vi "pan2txt.vi"(5 "seconds since 1Jan1904":timestamp, 6 "started":timestamp, 7 "stop button":refnum<vi>) -> ()   [LabVIEW 2010]
uses:
  Global 2.vi
panel:
  out "last mod":timestamp
  out "volume path":path
  out "Array":string[](array[string])
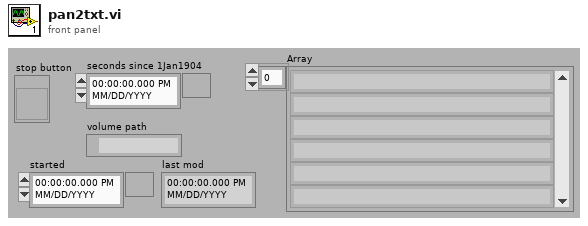
[diagram p1: front panel]
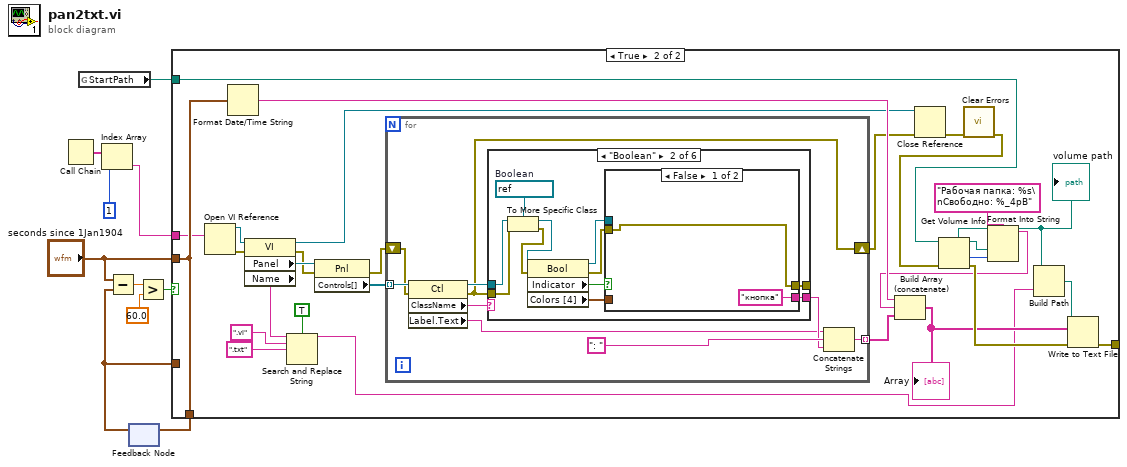
[diagram p0: block diagram]
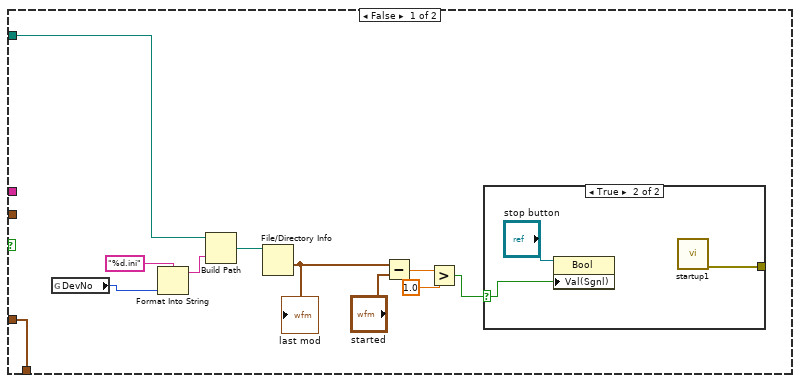
[diagram p2: hidden frame]
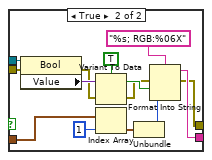
[diagram p5: hidden frame]
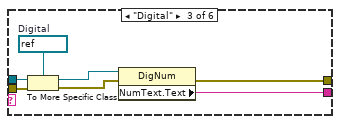
[diagram p6: hidden frame]
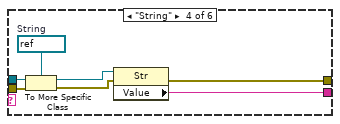
[diagram p7: hidden frame]
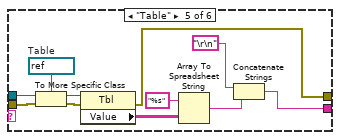
[diagram p8: hidden frame]
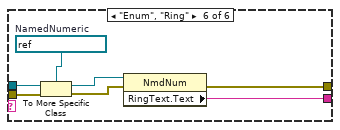
[diagram p9: hidden frame]
diagram:
  n1 = Call Chain() -> (call chain=w3:string[])
  n2 = global read "Global 2.vi" "StartPath"() -> (w1:path)
  n3 = Index Array(array=w3, index=1) -> (element=w2:string)
  n4 = feedback #1() -> (w5:timestamp)  [unwired: 1 in]
  n5 = Subtract(x="seconds since 1Jan1904", y=w5) -> (x-y=w10:dbl)
  n6 = Greater?(x=w10, y=60.0) -> (0:w8:bool)
  n7 = case shown="True" w8 {
    tunnel: "seconds since 1Jan1904" -> [_ w43]
    tunnel: [w21 w43] -> w6
    tunnel: w5 -> [w21 _]
    tunnel: [_ w41] -> _
    tunnel: w2 -> [_ w27]
    tunnel: w1 -> [w11 w25]
    frame False {
      n8 = global read "Global 2.vi" "DevNo"() -> (w20:i32)
      n9 = Format Into String(format string="%d.ini", w20) -> (resulting string=w18:string)  [unwired: 2 in, 1 out]
      n10 = Build Path(base path=w11, name or relative path=w18) -> (appended path=w17:path)
      n11 = File/Directory Info(path=w17) -> (last mod=w16:timestamp)  [unwired: 1 in, 6 out]
      "last mod" <- w16
      n12 = Subtract(x=w16, y="started") -> (x-y=w14:dbl)
      n13 = Greater?(x=w14, y=1.0) -> (0:w12:bool)
      n14 = case shown="True" w12 {
        selector: w12 -> [_ w23]
        tunnel: [_ w22] -> _
        frame False {
        }
        frame True {
          n15 = property class="Bool"(reference="stop button", "Val(Sgnl)"=w23) -> ()  [unwired: 1 in, 2 out]
          n16 = call "startup1.vi"() -> ("error out"=w22:errorcluster)  [unwired: 7 in]
        }
      }
    }
    frame True {
      n17 = Open VI Reference(vi path=w27) -> (vi reference=w50:refnum<vi>, error out=w53:errorcluster)  [unwired: 5 in]
      n18 = Format Date/Time String(seconds (now)=w43) -> (date/time string=w38:string)  [unwired: 2 in]
      n19 = property class="VI"(reference=w50, error in=w53) -> (reference out=w35:refnum<vi>, error out=w49:errorcluster, "Panel"=w52:refnum<vi>, "Name"=w32:string)
      n20 = Search and Replace String(case sensitive?=TRUE ("ignore case? (F)"), input string=w32, search string=".vi", replace string=".txt" ("replace string (\"\")")) -> (result string=w28:string)  [unwired: 4 in, 3 out]
      n21 = property class="Pnl"(reference=w52, error in=w49) -> (error out=w48:errorcluster, "Controls[]"=w51:refnum<vi>[])  [unwired: 1 out]
      n22 = for {
        tunnel: w51 -> [w62] mode=indexing
        tunnel: [w61] -> w44 mode=indexing
        shift-right: [w54] -> w36
        shift-left: w48 -> [w60]
        n23 = property class="Ctl"(reference=w62, error in=w60) -> (reference out=w57:refnum<vi>, error out=w54:errorcluster, "ClassName"=w58:string, "Label.Text"=w55:string)
        n24 = case shown="\"Boolean\"" w58 {
          selector: w58 -> [w64 _ _ _ _ _]
          tunnel: w57 -> [_ w75 w97 w104 w115 w122]
          tunnel: [w64 w73 w95 w102 w107 w120] -> w56
          tunnel: w54 -> [w63 w72 w94 w101 w111 w119]
          tunnel: [w63 w65 w92 w99 w106 w117] -> _
          frame "Any", Default {
          }
          frame "Boolean" {
            w74 = refnum<vi> refnum  # Boolean
            n25 = To More Specific Class(target class=w74, reference=w75, error in=w72) -> (specific class reference=w71:refnum<vi>, error out=w69:errorcluster)
            n26 = property class="Bool"(reference=w71, error in=w69) -> (reference out=w68:refnum<vi>, error out=w67:errorcluster, "Indicator"=w70:bool, "Colors [4]"=w66:cluster{u32, u32}[])
            n27 = case shown="False" w70 {
              tunnel: w68 -> [_ w91]
              tunnel: ["кнопка" w84] -> w73
              tunnel: w67 -> [w77 w82]
              tunnel: w66 -> [_ w81]
              tunnel: [w77 w80] -> w65
              frame False {
              }
              frame True {
                n28 = property class="Bool"(reference=w91, error in=w82) -> (error out=w79:errorcluster, "Value"=w88:variant)  [unwired: 1 out]
                n29 = Variant To Data(error in=w79, Variant=w88, type=TRUE) -> (error out=w78:errorcluster, data=w86:bool)
                n30 = Index Array(array=w81, index=1) -> (element=w90:cluster{u32, u32})
                n31 = Unbundle(w90) -> (w85:u32)  [unwired: 1 out]
                n32 = Format Into String(format string="%s; RGB:%06X", error in=w78, w86, w85) -> (resulting string=w84:string, error out=w80:errorcluster)  [unwired: 1 in]
              }
            }
          }
          frame "Digital" {
            w98 = refnum<vi> refnum  # Digital
            n33 = To More Specific Class(target class=w98, reference=w97, error in=w94) -> (specific class reference=w96:refnum<vi>, error out=w93:errorcluster)
            n34 = property class="DigNum"(reference=w96, error in=w93) -> (error out=w92:errorcluster, "NumText.Text"=w95:string)  [unwired: 1 out]
          }
          frame "String" {
            w105 = refnum<vi> refnum  # String
            n35 = To More Specific Class(target class=w105, reference=w104, error in=w101) -> (specific class reference=w103:refnum<vi>, error out=w100:errorcluster)
            n36 = property class="Str"(reference=w103, error in=w100) -> (error out=w99:errorcluster, "Value"=w102:string)  [unwired: 1 out]
          }
          frame "Table" {
            w116 = refnum<vi> refnum  # Table
            n37 = To More Specific Class(target class=w116, reference=w115, error in=w111) -> (specific class reference=w114:refnum<vi>, error out=w110:errorcluster)
            n38 = property class="Tbl"(reference=w114, error in=w110) -> (error out=w106:errorcluster, "Value"=w113:string[][])  [unwired: 1 out]
            n39 = Array To Spreadsheet String(array=w113, 3:"%s" ("format string")) -> (spreadsheet string=w109:string)  [unwired: 1 in]
            n40 = Concatenate Strings("\r\n", w109) -> (w107:string)
          }
          frame "Enum", "Ring" {
            w123 = refnum<vi> refnum  # NamedNumeric
            n41 = To More Specific Class(target class=w123, reference=w122, error in=w119) -> (specific class reference=w121:refnum<vi>, error out=w118:errorcluster)
            n42 = property class="NmdNum"(reference=w121, error in=w118) -> (error out=w117:errorcluster, "RingText.Text"=w120:string)  [unwired: 1 out]
          }
        }
        n43 = Concatenate Strings(w55, ": " ("string"), w56) -> (w61:string)
      }
      n44 = Close Reference(reference=w35, error in (no error)=w36) -> (error out=w34:errorcluster)
      n45 = call <vilib>:"Clear Errors.vi"("error in (no error)"=w34) -> ("error out"=w33:errorcluster)  [unwired: 6 in]
      n46 = Get Volume Info(8:w33, 11:w25) -> (0:w45:errorcluster, 1:w40:i64, 3:w26:path, 5:w47:path)  [unwired: 2 out]
      "volume path" <- w47
      n47 = Format Into String(format string="Рабочая папка: %s\nСвободно: %_4pB", w26, w40) -> (resulting string=w37:string)  [unwired: 2 in, 1 out]
      n48 = Build Array (concatenate)(w38, w37, w44) -> (w42:string[])
      "Array" <- w42
      n49 = Build Path(base path=w47, name or relative path=w28) -> (appended path=w46:path)
      n50 = Write to Text File(file (use dialog)=w46, text=w42, error in=w45) -> (error out=w41:errorcluster)  [unwired: 1 in, 2 out]
    }
  }
  n51 = feedback-in #1(w6) -> ()
